vi "GetEndpointChannelByAssetId.vi"(10 "asset id":string, 11 "channels in":T1[](array[typedef])) -> (1 "found":bool, 2 "channel":T1, 3 "channels out":T1[](array[typedef]))   [LabVIEW 2017, in "DeviceModelHelpers.lvlib"]
uses:
  <vilib>/addons/InsightCM/Utilities/DeviceModelHelpers/DeviceModelHelpers.lvlib
  <vilib>/addons/InsightCM/MessageBus/Base/controls/WirelessChannel.ctl
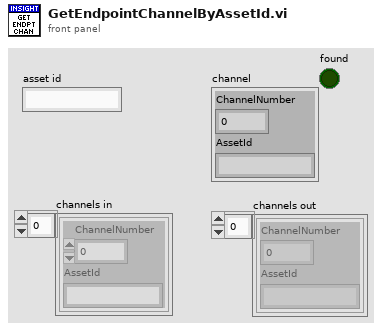
[diagram p1: front panel]
types:
  T1 = typedef "WirelessChannel.ctl" = cluster{"ChannelNumber":i32, "AssetId":string}
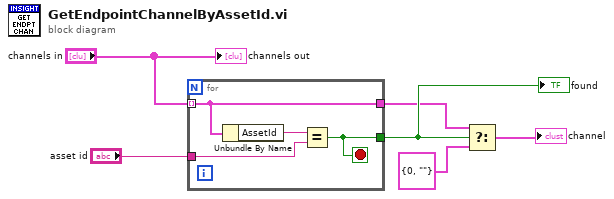
[diagram p0: block diagram]
diagram:
  n1 = for {
    tunnel: "channels in" -> [w10] mode=indexing
    tunnel: "asset id" -> [w8]
    tunnel: [w10] -> w3
    tunnel: [w7] -> w4
    stop <- w7 stop-if-true
    n2 = Unbundle By Name(w10) -> ("AssetId"=w9:string)
    n3 = Equal?(x=w9, y=w8) -> (x = y?=w7:bool)
  }
  "found" <- w4
  n4 = Select(t=w3, s=w4, f=T1 {"ChannelNumber"=0, "AssetId"=""}) -> (s? t:f=→"channel":T1)
  "channels out" <- "channels in"
